vi "Get Camera Data.vi"(8 "error in (no error)":errorcluster, 11 "Test Variables":T1={"Setpoint Function"=enum."Ramp", "Max Diam (mm)"=70.0, "Delay (sec)"=2.0, "T (sec)"=10.0, "Diastole (V)"=0.2, "Systole (V)"=0.5, "Inc Step (s)"=70.0}) -> (0 "error out":errorcluster, 1 "Diameter (mm)":dbl, 2 "Camera Buffer":u32, 3 "Camera Framerate":dbl, 5 "Stop?":bool)   [LabVIEW 2020]
uses:
  Controls/Test Variables.ctl
  Controls/Serpoint.ctl
  Controls/HW States.ctl
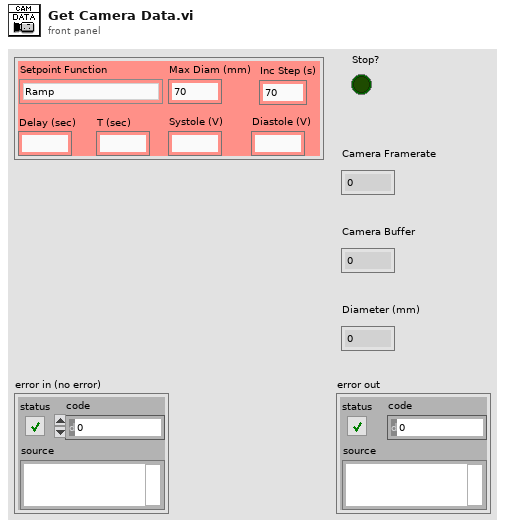
[diagram p1: front panel]
types:
  T1 = typedef "Test Variables.ctl" = cluster{"Setpoint Function":T2, "Max Diam (mm)":dbl, "Delay (sec)":dbl, "T (sec)":dbl, "Diastole (V)":dbl, "Systole (V)":dbl, "Inc Step (s)":dbl}
  T2 = typedef "Serpoint.ctl" = enum16{"Incremental PWM Step", "PWM Step", "Ramp", "Sinusoidal", "Blood-Pressure"}
  T3 = typedef "HW States.ctl" = enum16{"Initialize", "Input LED", "Input PWM", "Acquire Voltage", "Acquire Image", "Stop"}
  T4 = typedef "Camera output.ctl" = cluster{"Camera Framerate":dbl, "Camera Buffer":u32, "Diameter (mm)":dbl, "Image Out":T5, "Image Dst Out":T5}
  T5 = typedef "IMAQ Image.ctl" = refnum<image>
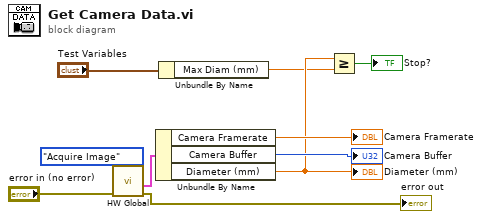
[diagram p0: block diagram]
diagram:
  n1 = call "HW Global.vi"("HW State"=HW_States."Acquire Image", "error in (no error)"="error in (no error)") -> ("error out"=→"error out":errorcluster, "Camera Data"=w8:T4)  [unwired: 6 in, 2 out]
  n2 = Unbundle By Name(w8) -> ("Camera Framerate"=→"Camera Framerate":dbl, "Camera Buffer"=→"Camera Buffer":u32, "Diameter (mm)"=w3:dbl)
  "Diameter (mm)" <- w3
  n3 = Unbundle By Name("Test Variables") -> ("Max Diam (mm)"=w2:dbl)
  n4 = Greater Or Equal?(x=w3, y=w2) -> (x >= y?=→"Stop?":bool)
